vi "PositionTactic_Init.vi"(0 "object in":refnum<class "PositionTactic.lvclass">, 5 "error in (no error)":errorcluster) -> (14 "object out":refnum<class "PositionTactic.lvclass">, 19 "error out":errorcluster)   [LabVIEW 2023, in "PositionTactic.lvclass"]
uses:
  PositionTactic.lvclass
  C:/Users/ebert/Documents/codes/SSL/repo/SSL_AI/NewSTP/NewTactics/Tactic_v2_class/Tactic_v2.lvclass
  NewSTP/NewSkills/GoToGuardPositionSkill_class/GoToGuardPositionSkill.lvclass
  C:/Users/ebert/Documents/codes/SSL/repo/SSL_AI/GoToSkill_v2_class/GoToSkill_v2.lvclass
  NewSTP/NewSkills/GoToTargetPositionSkill_class/GoToTargetPositionSkill.lvclass
  GoToSkill_v2_class/GoToSkill_v2.lvclass
  C:/Users/ebert/Documents/codes/SSL/repo/SSL_AI/NewSTP/NewSkills/Skill_v2_class/Skill_v2.lvclass
  NewSTP/NewTactics/Tactic_v2_class/Tactic_v2.lvclass
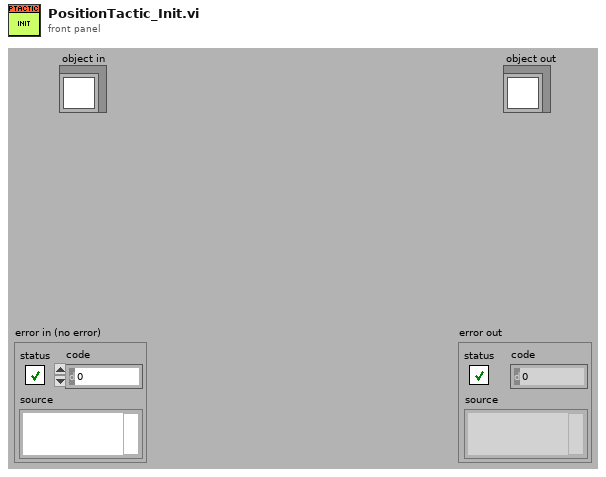
[diagram p1: front panel]
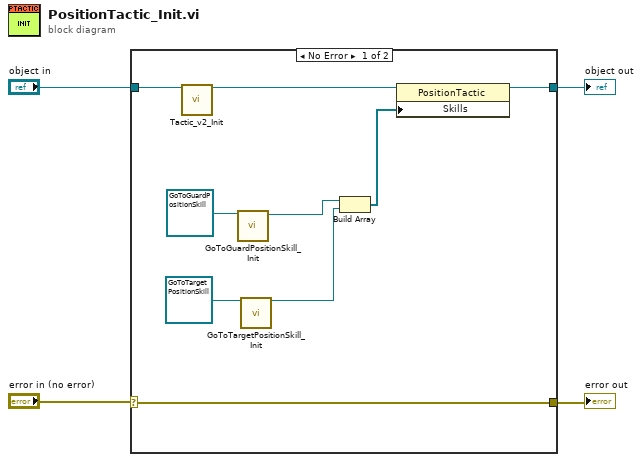
[diagram p0: block diagram]
diagram:
  n1 = case shown="No Error" "error in (no error)" {
    selector: "error in (no error)" -> [w13 w14]
    tunnel: "object in" -> [w12 w15]
    tunnel: [w9 w15] -> w3
    tunnel: [w13 w14] -> w1
    frame No Error {
      n2 = call "Tactic_v2_Init.vi"("object in"=w12) -> ("object out"=w11:refnum<class "PositionTactic.lvclass">)  [unwired: 17 in, 1 out]
      n3 = call "GoToGuardPositionSkill_Init.vi"("object in"=refnum<class "GoToGuardPositionSkill.lvclass"> refnum ("GoToGuardPositionSkill")) -> ("object out"=w6:refnum<class "GoToGuardPositionSkill.lvclass">)  [unwired: 17 in, 1 out]
      n4 = call "GoToTargetPositionSkill_Init.vi"("object in"=refnum<class "GoToTargetPositionSkill.lvclass"> refnum ("GoToGuardPositionSkill")) -> ("object out"=w5:refnum<class "GoToTargetPositionSkill.lvclass">)  [unwired: 17 in, 1 out]
      n5 = Build Array(w6, w5) -> (w10:refnum<class "GoToSkill_v2.lvclass">[])
      n6 = property class="PositionTactic"(reference=w11, "Skills"=w10) -> (reference out=w9:refnum<class "PositionTactic.lvclass">)  [unwired: 1 in, 1 out]
    }
    frame Error {
    }
  }
  "object out" <- w3
  "error out" <- w1
